vi "Convert CAN Frame.vi"(8 "error in (no error)":errorcluster, 9 "timestamp":timestamp, 10 "CAN frame":T1 {"type" items=["CAN Data", "CAN Remote"]; "identifier" format="%.0x"}, 11 "tdms file":refnum<k34>) -> (0 "error out":errorcluster, 3 "tdms file out":refnum<k34>)   [LabVIEW 2014]
uses:
  <vilib>/RioEmbeddedCAN/RioEmbeddedCAN.llb/CANFrameControl.ctl
  TDMS Timestamp and Data Double.vi
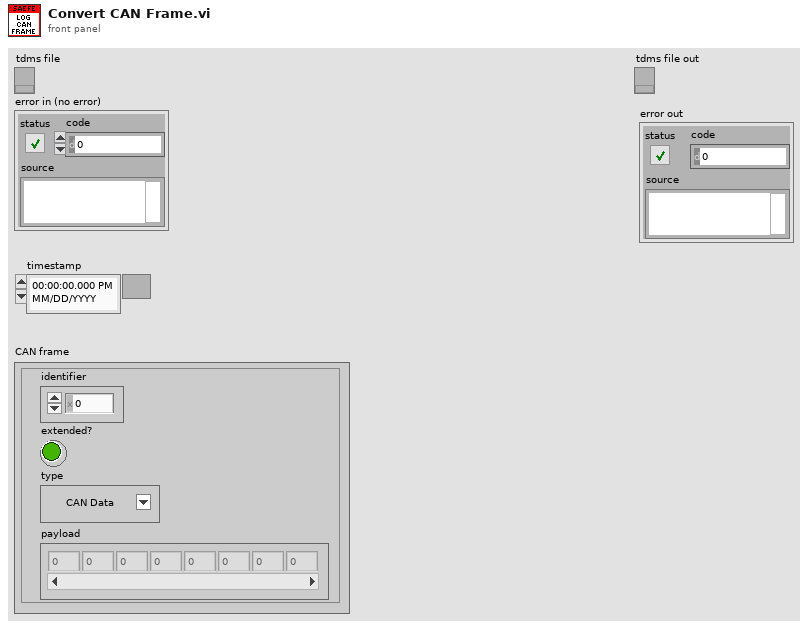
[diagram p1: front panel]
types:
  T1 = typedef "CANFrameControl.ctl" = cluster{"identifier":u32, "extended?":bool, "type":u8, "payload":u8[]}
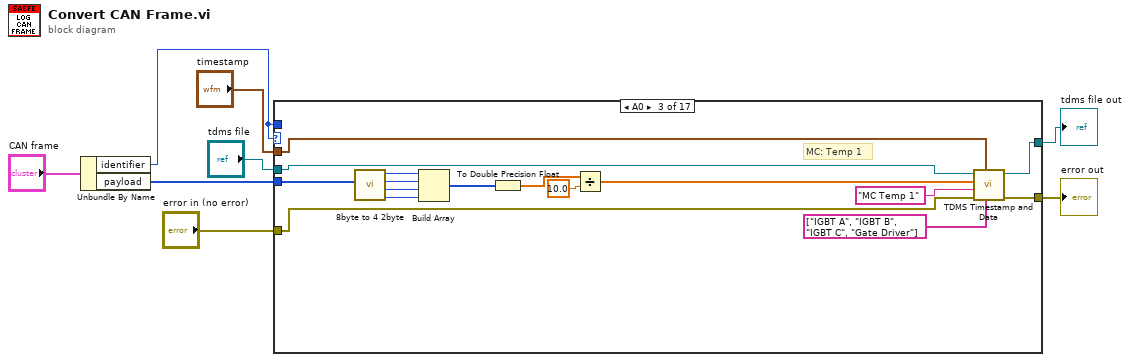
[diagram p0: block diagram]
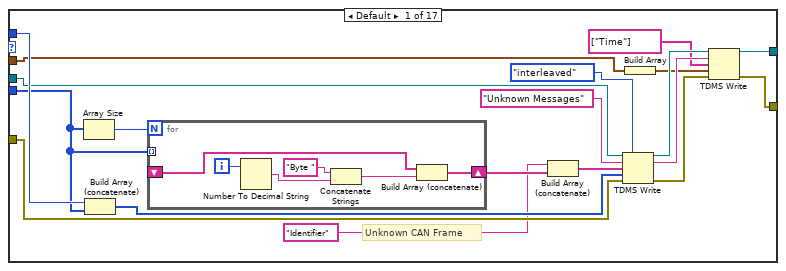
[diagram p2: hidden frame]
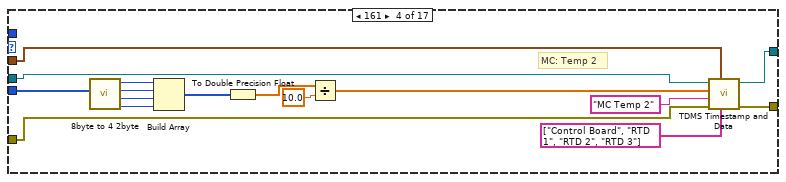
[diagram p4: hidden frame]
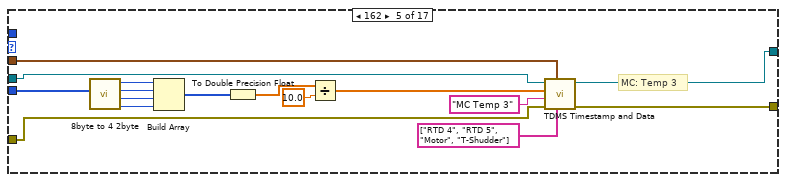
[diagram p5: hidden frame]
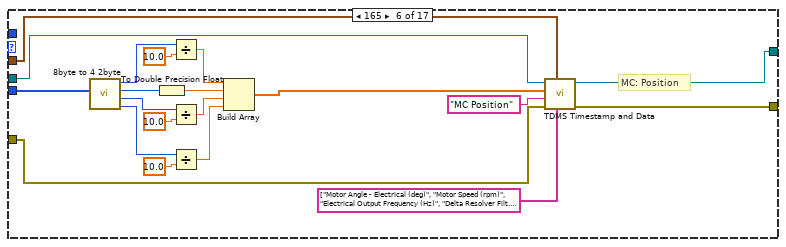
[diagram p6: hidden frame]
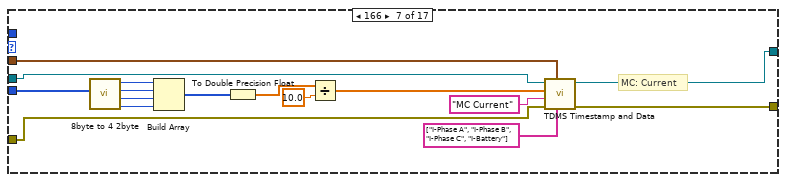
[diagram p7: hidden frame]
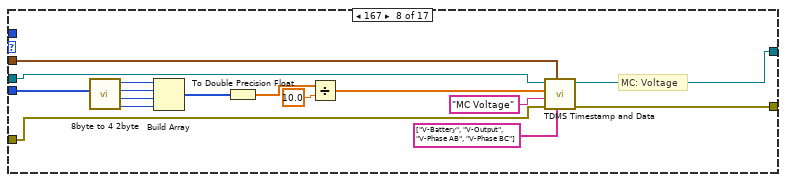
[diagram p8: hidden frame]
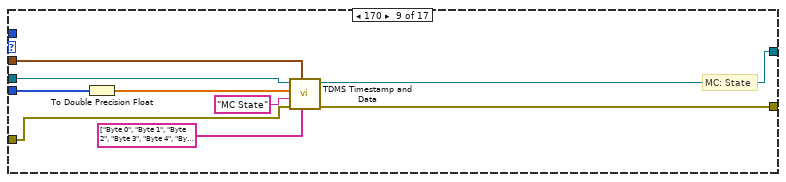
[diagram p9: hidden frame]
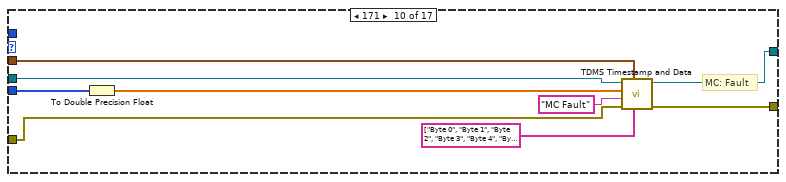
[diagram p10: hidden frame]
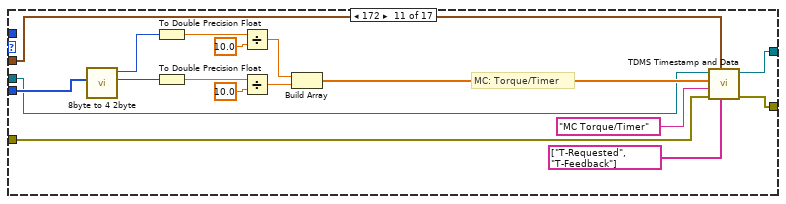
[diagram p11: hidden frame]
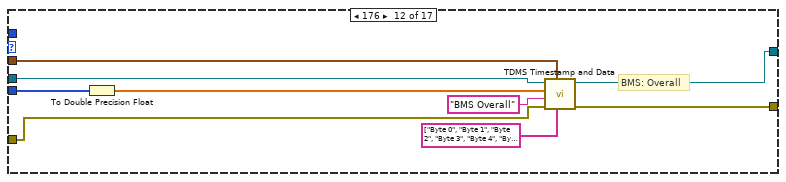
[diagram p12: hidden frame]
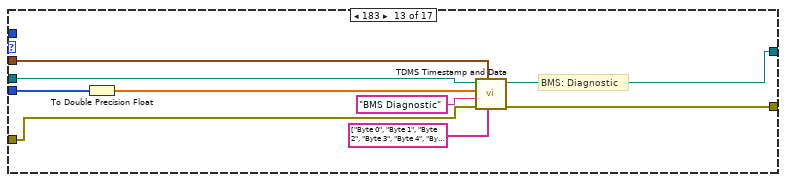
[diagram p13: hidden frame]
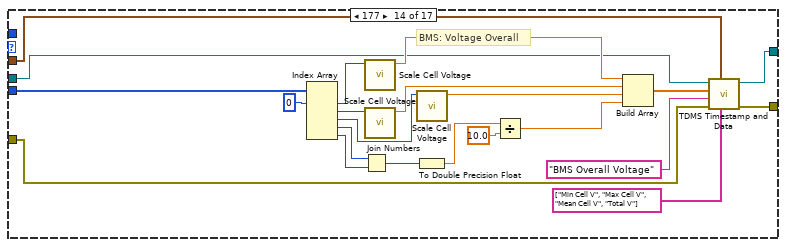
[diagram p14: hidden frame]
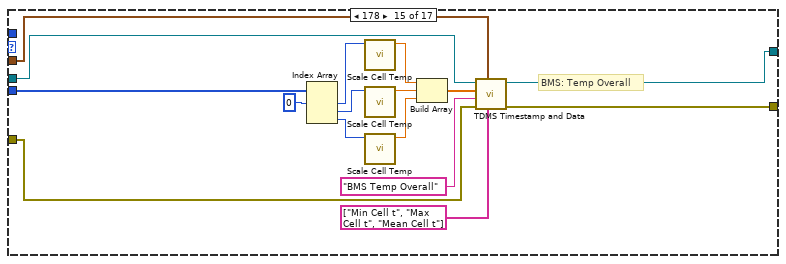
[diagram p15: hidden frame]
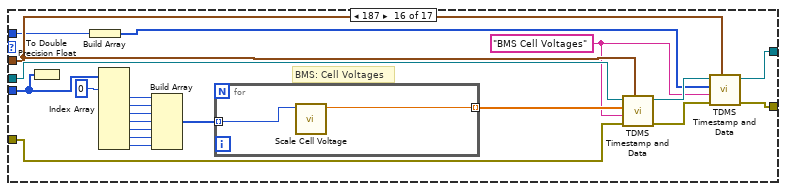
[diagram p16: hidden frame]
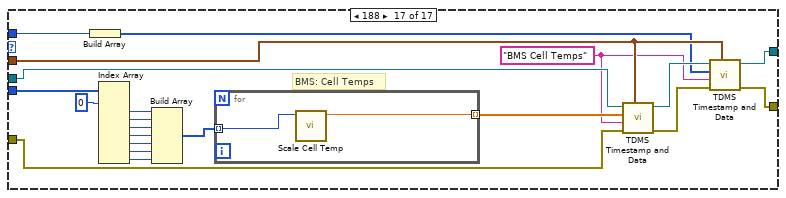
[diagram p17: hidden frame]
diagram:
  n1 = Unbundle By Name("CAN frame") -> ("identifier"=w5:u32, "payload"=w7:u8[])
  n2 = case shown="A0" w5 {
    tunnel: w5 -> [w27 _ _ _ _ _ _ _ _ _ _ _ _ _ _ w231 w251]
    tunnel: w7 -> [w9 _ w51 w67 w83 w103 w119 w135 w144 w153 w170 w176 w185 w210 w226 w236 w259]
    tunnel: "timestamp" -> [w14 _ w37 w59 w73 w91 w109 w124 w143 w150 w159 w177 w186 w193 w221 w232 w253]
    tunnel: "tdms file" -> [w26 w35 w43 w58 w74 w90 w111 w127 w142 w151 w160 w179 w188 w195 w220 w238 w261]
    tunnel: [w11 w35 w40 w55 w71 w87 w105 w122 w139 w147 w156 w173 w182 w191 w212 w228 w255] -> w3
    tunnel: "error in (no error)" -> [w25 w34 w36 w57 w72 w89 w110 w126 w141 w149 w158 w178 w187 w194 w219 w237 w260]
    tunnel: [w12 w34 w39 w56 w70 w88 w104 w121 w138 w146 w155 w172 w181 w190 w211 w227 w254] -> w1
    frame Default {
      # "Unknown CAN Frame"
      n3 = Array Size(array=w9) -> (size(s)=w10:i32)
      n4 = Build Array (concatenate)(w27, w9) -> (w24:u32[])
      n5 = for {
        N: w10 -> [_]
        tunnel: w9 -> [_] mode=indexing
        shift-right: [w32] -> w23
        shift-left: _ -> [w28]
        i -> [w31]
        n6 = Number To Decimal String(number=w31) -> (decimal integer string=w30:string)  [unwired: 1 in]
        n7 = Concatenate Strings("Byte " ("string"), w30) -> (w33:string)
        n8 = Build Array (concatenate)(w28, w33) -> (w32:string[])
      }
      n9 = Build Array (concatenate)("Identifier", w23) -> (w21:string[])
      n10 = TDMS Write(0:w26, 1:enum16{"decimated", "interleaved"}."interleaved" ("data layout (0:decimated)"), 5:"Unknown Messages" ("group name in (Untitled)"), 7:w21, 9:w24, 11:w25) -> (4:w18:refnum<k34>, 6:w16:string, 15:w17:errorcluster)  [unwired: 1 out]
      n11 = Build Array(w14) -> (w13:timestamp[])
      n12 = TDMS Write(0:w18, 5:w16, 7:string[] ["Time"] ("channel name(s) in (Untitled)"), 9:w13, 11:w17) -> (4:w11:refnum<k34>, 15:w12:errorcluster)  [unwired: 1 in, 2 out]
    }
    frame 0 {
      # "Do nothing for NULL frame"
    }
    frame 160 {
      # "MC: Temp 1"
      n13 = call "8byte to 4 2byte.vi"("payload"=w51) -> ("7,6"=w47:u16, "5,4"=w48:u16, "3,2"=w49:u16, "1,0"=w50:u16)  [unwired: 7 in]
      n14 = Build Array(w50, w49, w48, w47) -> (w44:u16[])
      n15 = To Double Precision Float(number=w44) -> (double precision float=w45:dbl[])
      n16 = Divide(x=w45, y=10.0) -> (x/y=w38:dbl[])
      n17 = call-poly "TDMS Timestamp and Data.vi"("channel name(s) in (Untitled)"=string[] ["IGBT A", "IGBT B", "IGBT C", "Gate Driver"], "timestamp"=w37, "error in (no error)"=w36, "group name in (Untitled)"="MC Temp 1", "Array"=w38, "Refnum in"=w43) -> ("error out"=w39:errorcluster, "Refnum out"=w40:refnum<k34>)  [unwired: 4 in]
    }
    frame 161 {
      # "MC: Temp 2"
      n18 = call "8byte to 4 2byte.vi"("payload"=w67) -> ("7,6"=w63:u16, "5,4"=w64:u16, "3,2"=w65:u16, "1,0"=w66:u16)  [unwired: 7 in]
      n19 = Build Array(w66, w65, w64, w63) -> (w60:u16[])
      n20 = To Double Precision Float(number=w60) -> (double precision float=w61:dbl[])
      n21 = Divide(x=w61, y=10.0) -> (x/y=w54:dbl[])
      n22 = call-poly "TDMS Timestamp and Data.vi"("channel name(s) in (Untitled)"=string[] ["Control Board", "RTD 1", "RTD 2", "RTD 3"], "timestamp"=w59, "error in (no error)"=w57, "group name in (Untitled)"="MC Temp 2", "Array"=w54, "Refnum in"=w58) -> ("error out"=w56:errorcluster, "Refnum out"=w55:refnum<k34>)  [unwired: 4 in]
    }
    frame 162 {
      # "MC: Temp 3"
      n23 = call "8byte to 4 2byte.vi"("payload"=w83) -> ("7,6"=w79:u16, "5,4"=w80:u16, "3,2"=w81:u16, "1,0"=w82:u16)  [unwired: 7 in]
      n24 = Build Array(w82, w81, w80, w79) -> (w76:u16[])
      n25 = To Double Precision Float(number=w76) -> (double precision float=w77:dbl[])
      n26 = Divide(x=w77, y=10.0) -> (x/y=w75:dbl[])
      n27 = call-poly "TDMS Timestamp and Data.vi"("channel name(s) in (Untitled)"=string[] ["RTD 4", "RTD 5", "Motor", "T-Shudder"], "timestamp"=w73, "error in (no error)"=w72, "group name in (Untitled)"="MC Temp 3", "Array"=w75, "Refnum in"=w74) -> ("error out"=w70:errorcluster, "Refnum out"=w71:refnum<k34>)  [unwired: 4 in]
    }
    frame 165 {
      # "MC: Position"
      n28 = call "8byte to 4 2byte.vi"("payload"=w103) -> ("7,6"=w98:u16, "5,4"=w99:u16, "3,2"=w93:u16, "1,0"=w102:u16)  [unwired: 7 in]
      n29 = To Double Precision Float(number=w93) -> (double precision float=w92:dbl)
      n30 = Divide(x=w102, y=10.0) -> (x/y=w97:dbl)
      n31 = Divide(x=w99, y=10.0) -> (x/y=w96:dbl)
      n32 = Divide(x=w98, y=10.0) -> (x/y=w95:dbl)
      n33 = Build Array(w97, w92, w96, w95) -> (w84:dbl[])
      n34 = call-poly "TDMS Timestamp and Data.vi"("channel name(s) in (Untitled)"=string[] ["Motor Angle - Electrical (deg)", "Motor Speed (rpm)", "Electrical Output Frequency (Hz)", "Delta Resolver Filt. (deg)"], "timestamp"=w91, "error in (no error)"=w89, "group name in (Untitled)"="MC Position", "Array"=w84, "Refnum in"=w90) -> ("error out"=w88:errorcluster, "Refnum out"=w87:refnum<k34>)  [unwired: 4 in]
    }
    frame 166 {
      # "MC: Current"
      n35 = call "8byte to 4 2byte.vi"("payload"=w119) -> ("7,6"=w115:u16, "5,4"=w116:u16, "3,2"=w117:u16, "1,0"=w118:u16)  [unwired: 7 in]
      n36 = Build Array(w118, w117, w116, w115) -> (w112:u16[])
      n37 = To Double Precision Float(number=w112) -> (double precision float=w113:dbl[])
      n38 = Divide(x=w113, y=10.0) -> (x/y=w108:dbl[])
      n39 = call-poly "TDMS Timestamp and Data.vi"("channel name(s) in (Untitled)"=string[] ["I-Phase A", "I-Phase B", "I-Phase C", "I-Battery"], "timestamp"=w109, "error in (no error)"=w110, "group name in (Untitled)"="MC Current", "Array"=w108, "Refnum in"=w111) -> ("error out"=w104:errorcluster, "Refnum out"=w105:refnum<k34>)  [unwired: 4 in]
    }
    frame 167 {
      # "MC: Voltage"
      n40 = call "8byte to 4 2byte.vi"("payload"=w135) -> ("7,6"=w131:u16, "5,4"=w132:u16, "3,2"=w133:u16, "1,0"=w134:u16)  [unwired: 7 in]
      n41 = Build Array(w134, w133, w132, w131) -> (w128:u16[])
      n42 = To Double Precision Float(number=w128) -> (double precision float=w129:dbl[])
      n43 = Divide(x=w129, y=10.0) -> (x/y=w125:dbl[])
      n44 = call-poly "TDMS Timestamp and Data.vi"("channel name(s) in (Untitled)"=string[] ["V-Battery", "V-Output", "V-Phase AB", "V-Phase BC"], "timestamp"=w124, "error in (no error)"=w126, "group name in (Untitled)"="MC Voltage", "Array"=w125, "Refnum in"=w127) -> ("error out"=w121:errorcluster, "Refnum out"=w122:refnum<k34>)  [unwired: 4 in]
    }
    frame 170 {
      # "MC: State"
      n45 = To Double Precision Float(number=w144) -> (double precision float=w140:dbl[])
      n46 = call-poly "TDMS Timestamp and Data.vi"("channel name(s) in (Untitled)"=string[] ["Byte 0", "Byte 1", "Byte 2", "Byte 3", "Byte 4", "Byte 5", "Byte 6", "Byte 7"], "timestamp"=w143, "error in (no error)"=w141, "group name in (Untitled)"="MC State", "Array"=w140, "Refnum in"=w142) -> ("error out"=w138:errorcluster, "Refnum out"=w139:refnum<k34>)  [unwired: 4 in]
    }
    frame 171 {
      # "MC: Fault"
      n47 = To Double Precision Float(number=w153) -> (double precision float=w152:dbl[])
      n48 = call-poly "TDMS Timestamp and Data.vi"("channel name(s) in (Untitled)"=string[] ["Byte 0", "Byte 1", "Byte 2", "Byte 3", "Byte 4", "Byte 5", "Byte 6", "Byte 7"], "timestamp"=w150, "error in (no error)"=w149, "group name in (Untitled)"="MC Fault", "Array"=w152, "Refnum in"=w151) -> ("error out"=w146:errorcluster, "Refnum out"=w147:refnum<k34>)  [unwired: 4 in]
    }
    frame 172 {
      # "MC: Torque/Timer"
      n49 = call "8byte to 4 2byte.vi"("payload"=w170) -> ("3,2"=w166:u16, "1,0"=w169:u16)  [unwired: 7 in, 2 out]
      n50 = To Double Precision Float(number=w169) -> (double precision float=w168:dbl)
      n51 = To Double Precision Float(number=w166) -> (double precision float=w165:dbl)
      n52 = Divide(x=w168, y=10.0) -> (x/y=w163:dbl)
      n53 = Divide(x=w165, y=10.0) -> (x/y=w162:dbl)
      n54 = Build Array(w163, w162) -> (w161:dbl[])
      n55 = call-poly "TDMS Timestamp and Data.vi"("channel name(s) in (Untitled)"=string[] ["T-Requested", "T-Feedback"], "timestamp"=w159, "error in (no error)"=w158, "group name in (Untitled)"="MC Torque/Timer", "Array"=w161, "Refnum in"=w160) -> ("error out"=w155:errorcluster, "Refnum out"=w156:refnum<k34>)  [unwired: 4 in]
    }
    frame 176 {
      # "BMS: Overall"
      n56 = To Double Precision Float(number=w176) -> (double precision float=w175:dbl[])
      n57 = call-poly "TDMS Timestamp and Data.vi"("channel name(s) in (Untitled)"=string[] ["Byte 0", "Byte 1", "Byte 2", "Byte 3", "Byte 4", "Byte 5", "Byte 6", "Byte 7"], "timestamp"=w177, "error in (no error)"=w178, "group name in (Untitled)"="BMS Overall", "Array"=w175, "Refnum in"=w179) -> ("error out"=w172:errorcluster, "Refnum out"=w173:refnum<k34>)  [unwired: 4 in]
    }
    frame 183 {
      # "BMS: Diagnostic"
      n58 = To Double Precision Float(number=w185) -> (double precision float=w184:dbl[])
      n59 = call-poly "TDMS Timestamp and Data.vi"("channel name(s) in (Untitled)"=string[] ["Byte 0", "Byte 1", "Byte 2", "Byte 3", "Byte 4", "Byte 5", "Byte 6", "Byte 7"], "timestamp"=w186, "error in (no error)"=w187, "group name in (Untitled)"="BMS Diagnostic", "Array"=w184, "Refnum in"=w188) -> ("error out"=w181:errorcluster, "Refnum out"=w182:refnum<k34>)  [unwired: 4 in]
    }
    frame 177 {
      # "BMS: Voltage Overall"
      n60 = Index Array(array=w210, index #1=0 ("index")) -> (element #1=w208:u8, element #2=w207:u8, element #3=w206:u8, element #4=w205:u8, element #5=w204:u8)  [unwired: 4 in]
      n61 = Join Numbers(hi=w205, lo=w204) -> ((hi.lo)=w203:u16)
      n62 = call "Scale Cell Voltage.vi"("Numeric in"=w208) -> ("Numeric out"=w200:dbl)  [unwired: 10 in]
      n63 = call "Scale Cell Voltage.vi"("Numeric in"=w207) -> ("Numeric out"=w199:dbl)  [unwired: 10 in]
      n64 = call "Scale Cell Voltage.vi"("Numeric in"=w206) -> ("Numeric out"=w198:dbl)  [unwired: 10 in]
      n65 = To Double Precision Float(number=w203) -> (double precision float=w202:dbl)
      n66 = Divide(x=w202, y=10.0) -> (x/y=w197:dbl)
      n67 = Build Array(w200, w199, w198, w197) -> (w196:dbl[])
      n68 = call-poly "TDMS Timestamp and Data.vi"("channel name(s) in (Untitled)"=string[] ["Min Cell V", "Max Cell V", "Mean Cell V", "Total V"], "timestamp"=w193, "error in (no error)"=w194, "group name in (Untitled)"="BMS Overall Voltage", "Array"=w196, "Refnum in"=w195) -> ("error out"=w190:errorcluster, "Refnum out"=w191:refnum<k34>)  [unwired: 4 in]
    }
    frame 178 {
      # "BMS: Temp Overall"
      n69 = Index Array(array=w226, index #1=0 ("index")) -> (element #1=w224:u8, element #2=w223:u8, element #3=w222:u8)  [unwired: 2 in]
      n70 = call "Scale Cell Temp.vi"("Numeric in"=w224) -> ("Numeric out"=w218:dbl)  [unwired: 10 in]
      n71 = call "Scale Cell Temp.vi"("Numeric in"=w223) -> ("Numeric out"=w217:dbl)  [unwired: 10 in]
      n72 = call "Scale Cell Temp.vi"("Numeric in"=w222) -> ("Numeric out"=w216:dbl)  [unwired: 10 in]
      n73 = Build Array(w218, w217, w216) -> (w215:dbl[])
      n74 = call-poly "TDMS Timestamp and Data.vi"("channel name(s) in (Untitled)"=string[] ["Min Cell t", "Max Cell t", "Mean Cell t"], "timestamp"=w221, "error in (no error)"=w219, "group name in (Untitled)"="BMS Temp Overall", "Array"=w215, "Refnum in"=w220) -> ("error out"=w211:errorcluster, "Refnum out"=w212:refnum<k34>)  [unwired: 4 in]
    }
    frame 187 {
      w229 = "BMS Cell Voltages" ("group name in (Untitled)")
      # "BMS: Cell Voltages"
      n75 = To Double Precision Float(number=w236) -> ()  [unwired: 1 out]
      n76 = Build Array(w231) -> (w230:u32[])
      n77 = Index Array(array=w236, index #1=0 ("index")) -> (element #2=w246:u8, element #3=w245:u8, element #4=w244:u8, element #5=w243:u8, element #6=w242:u8, element #7=w241:u8, element #8=w240:u8)  [unwired: 7 in, 1 out]
      n78 = Build Array(w246, w245, w244, w243, w242, w241, w240) -> (w239:u8[])
      n79 = for {
        tunnel: w239 -> [w249] mode=indexing
        tunnel: [w248] -> w235 mode=indexing
        n80 = call "Scale Cell Voltage.vi"("Numeric in"=w249) -> ("Numeric out"=w248:dbl)  [unwired: 10 in]
      }
      n81 = call-poly "TDMS Timestamp and Data.vi"("timestamp"=w232, "error in (no error)"=w237, "group name in (Untitled)"=w229, "Array"=w235, "Refnum in"=w238) -> ("error out"=w233:errorcluster, "Refnum out"=w234:refnum<k34>)  [unwired: 5 in]
      n82 = call-poly "TDMS Timestamp and Data.vi"("timestamp"=w232, "error in (no error)"=w233, "group name in (Untitled)"=w229, "Array"=w230, "Refnum in"=w234) -> ("error out"=w227:errorcluster, "Refnum out"=w228:refnum<k34>)  [unwired: 5 in]
    }
    frame 188 {
      w252 = "BMS Cell Temps" ("group name in (Untitled)")
      # "BMS: Cell Temps"
      n83 = Build Array(w251) -> (w250:u32[])
      n84 = Index Array(array=w259, index #1=0 ("index")) -> (element #2=w269:u8, element #3=w268:u8, element #4=w267:u8, element #5=w266:u8, element #6=w265:u8, element #7=w264:u8, element #8=w263:u8)  [unwired: 7 in, 1 out]
      n85 = Build Array(w269, w268, w267, w266, w265, w264, w263) -> (w262:u8[])
      n86 = for {
        tunnel: w262 -> [w271] mode=indexing
        tunnel: [w272] -> w258 mode=indexing
        n87 = call "Scale Cell Temp.vi"("Numeric in"=w271) -> ("Numeric out"=w272:dbl)  [unwired: 10 in]
      }
      n88 = call-poly "TDMS Timestamp and Data.vi"("timestamp"=w253, "error in (no error)"=w260, "group name in (Untitled)"=w252, "Array"=w258, "Refnum in"=w261) -> ("error out"=w256:errorcluster, "Refnum out"=w257:refnum<k34>)  [unwired: 5 in]
      n89 = call-poly "TDMS Timestamp and Data.vi"("timestamp"=w253, "error in (no error)"=w256, "group name in (Untitled)"=w252, "Array"=w250, "Refnum in"=w257) -> ("error out"=w254:errorcluster, "Refnum out"=w255:refnum<k34>)  [unwired: 5 in]
    }
  }
  "tdms file out" <- w3
  "error out" <- w1
